vi "Logging Stopped.vi"(8 "error in (no error)":errorcluster, 11 "Data Logger Actor Reply Interface in":refnum<class "Data Logger Actor Reply Interface.lvclass">) -> (0 "error out":errorcluster, 3 "Data Logger Actor Reply Interface out":refnum<class "Data Logger Actor Reply Interface.lvclass">)   [LabVIEW 2024, in "Data Logger Actor Reply Interface.lvlib" / "Data Logger Actor Reply Interface.lvclass"]
uses:
  Data Logger Actor Reply Interface.lvclass
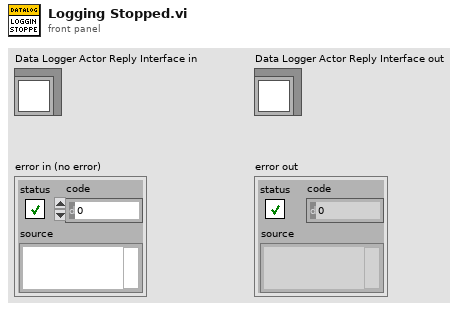
[diagram p1: front panel]
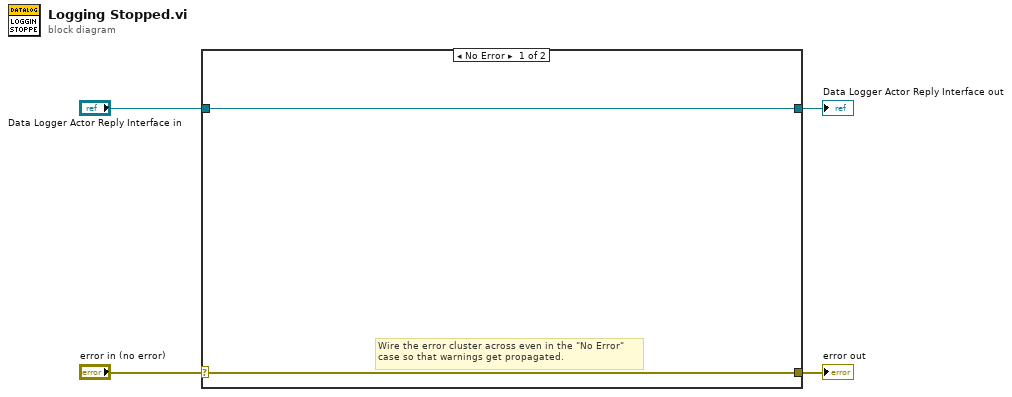
[diagram p0: block diagram]
diagram:
  n1 = case shown="No Error" "error in (no error)" {
    selector: "error in (no error)" -> [w5 w8]
    tunnel: [w5 w8] -> w3
    tunnel: [w6 w7] -> w1
    tunnel: "Data Logger Actor Reply Interface in" -> [w6 w7]
    frame No Error {
      # "Wire the error cluster across even in the \"No Error\"\ncase so that warnings get propagated."
    }
    frame Error {
    }
  }
  "error out" <- w3
  "Data Logger Actor Reply Interface out" <- w1
